vi "pid-toolkit.vi"() -> ()   [LabVIEW 2018, in "pid-toolkit.lvlib"]
uses:
  pid-toolkit.lvlib
  <vilib>/addons/control/pid/autopid.llb/PID autotuning parameters (FO).ctl
  <vilib>/Platform/TimedLoop/XDataNode/timing_clust.ctl
  <vilib>/Platform/TimedLoop/XDataNode/nitl_modes.ctl
  <vilib>/Platform/TimedLoop/XDataNode/wakeup.ctl
  <vilib>/addons/control/pid/pid.llb/PID Advanced (DBL).vi
  <vilib>/platform/TimedLoop/XDataNode/XDataNode.xnode
  <vilib>/Platform/TimedLoop/XDataNode/XDNodeRunTimeDep.lvlib
  <vilib>/addons/control/pid/NI_PID_autopid.lvlib
  <vilib>/addons/control/pid/NI_PID_pid.lvlib
panel:
  out "General Error":errorcluster
  out "Plot":T1(graph)
  out "tuning completed?":bool
  out "plant parameters out":T2={"process gain"=1.0, "time constant (s)"=0.01, "delay time (s)"=0.0} {"delay time (s)" format="%.3f"; "time constant (s)" format="%.3f"; "process gain" format="%.3f"}
  out "PID gains out":T3={"proportional gain (Kc)"=1.0, "integral time (Ti, min)"=0.01, "derivative time (Td, min)"=0.0} {"derivative time (Td, min)" format="%.3f"; "integral time (Ti, min)" format="%.3f"; "proportional gain (Kc)" format="%.3f"}
  in  "reinitialize? (F)":bool
  in  "plant parameters in":T2={"process gain"=1.0, "time constant (s)"=0.01, "delay time (s)"=0.0} {"delay time (s)" format="%.3f"; "time constant (s)" format="%.3f"; "process gain" format="%.3f"}
  in  "PID gains in":T3={"proportional gain (Kc)"=1.0, "integral time (Ti, min)"=0.01, "derivative time (Td, min)"=0.0} {"derivative time (Td, min)" format="%.3f"; "integral time (Ti, min)" format="%.3f"; "proportional gain (Kc)" format="%.3f"}
  in  "output range":cluster{"output high":dbl, "output low":dbl}={"output high"=100.0, "output low"=-100.0} {"output low" format="%.2f"; "output high" format="%.2f"}
  in  "desired temperature":dbl format="%.2f"
  in  "beta":dbl=1.0 format="%.2f"
  in  "autotuning parameters":T4={"type of controller"=0, "time constant factor"=2.0, "step amplitude"=1.0} {"step amplitude" format="%.2f"; "type of controller" items=["P", "PI", "PID"]}
  in  "autotune? (F)":bool
  in  "auto? (T)":bool=TRUE
  in  "alpha":dbl=0.1 format="%.2f"
  out "Output unfiltered":dbl format="%.2f"
  out "Output":u16
  out "High":bool
  out "Low":bool
  in  "Manual":u8(slide) scale=0.0..255.0
  out "Modbus Error":errorcluster
  in  "Off Hook":bool
  in  "Update Rate":dbl caption="Rate"
  out "Failure":bool
  out "Updating":bool
  in  "Update Now":bool
  in  "Maximum":sgl
  in  "Minimum":sgl
  out "Thermometer":sgl(slide) scale=0.0..260.0
  in  "Force exit out of loop":bool
  out "Interval":i64
  out "Duration":i64
  out "Cycle":i32
  in  "Frequency":dbl(slide) scale=0.1..10.0
  # "Loop"
  # "Modbus"
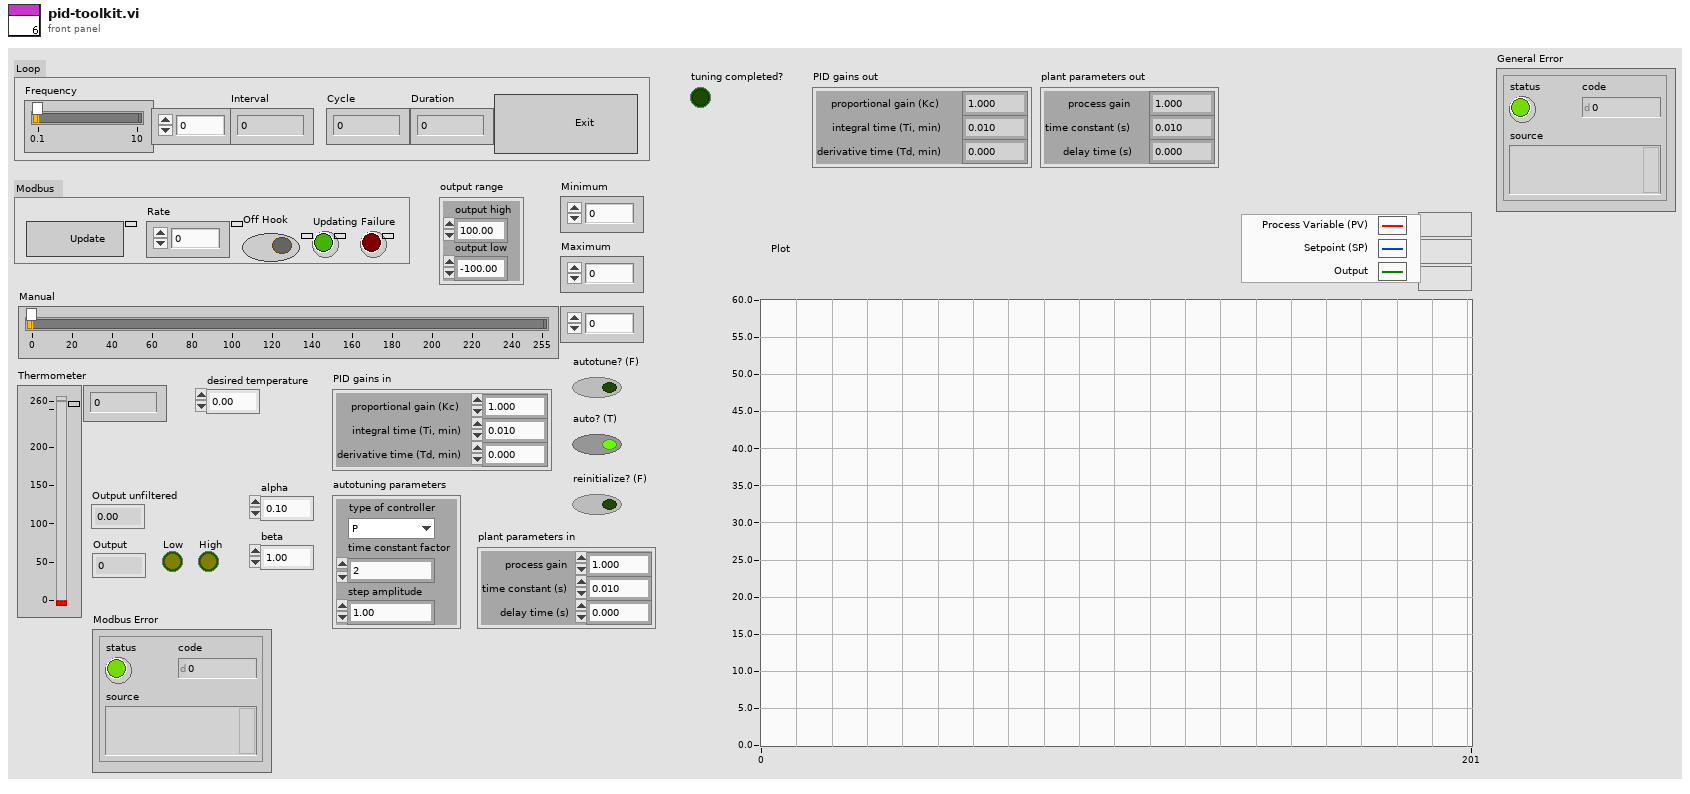
[diagram p1: front panel]
types:
  T1 = cluster{dbl, "desired temperature":dbl, "output":dbl}
  T2 = cluster{"process gain":dbl, "time constant (s)":dbl, "delay time (s)":dbl}
  T3 = cluster{"proportional gain (Kc)":dbl, "integral time (Ti, min)":dbl, "derivative time (Td, min)":dbl}
  T4 = typedef "NI_PID_autopid.lvlib/PID autotuning parameters (FO).ctl" = cluster{"type of controller":u16, "time constant factor":dbl, "step amplitude":dbl}
  T5 = typedef "XDNodeRunTimeDep.lvlib/timing_clust.ctl" = cluster{"Expected End [f-1]":u64, "Actual End [f-1]":u64, "Finished Late? [f-1]":bool, "Expected End [i-1]":u64, "Actual End [i-1]":u64, "Finished Late? [i-1]":bool, "Expected Start [i]":u64, "Actual Start [i]":u64, "Expected Start [f]":u64, "Actual Start [f]":u64, "Source Name":string, "Structure Name":string, "Period":i64, "Deadline":i64, "Offset":i64, "Start":i64, "Priority":i32, "Timeout":i32, "Mode":T6, "Wakeup Reason":T7, "Error":errorcluster, "Source Type":string, "Secondary Source Type":string, "Global End Time":u64, "Global Start Time":u64, "Frame Duration":u64, "Iteration Duration":u64, "Assigned CPU":i32, "I/O Scan Engine Mode":u32}
  T6 = typedef "XDNodeRunTimeDep.lvlib/nitl_modes.ctl" = enum32{"No Change", "Process missed periods, maintain original phase", "Discard missed periods, maintain original phase", "Process missed periods, ignore original phase", "Discard missed periods, ignore original phase"}
  T7 = typedef "XDNodeRunTimeDep.lvlib/wakeup.ctl" = enum32{"Normal", "Aborted", "Asynchronous wakeup", "Timing source error", "Timed loop error", "Timeout"}
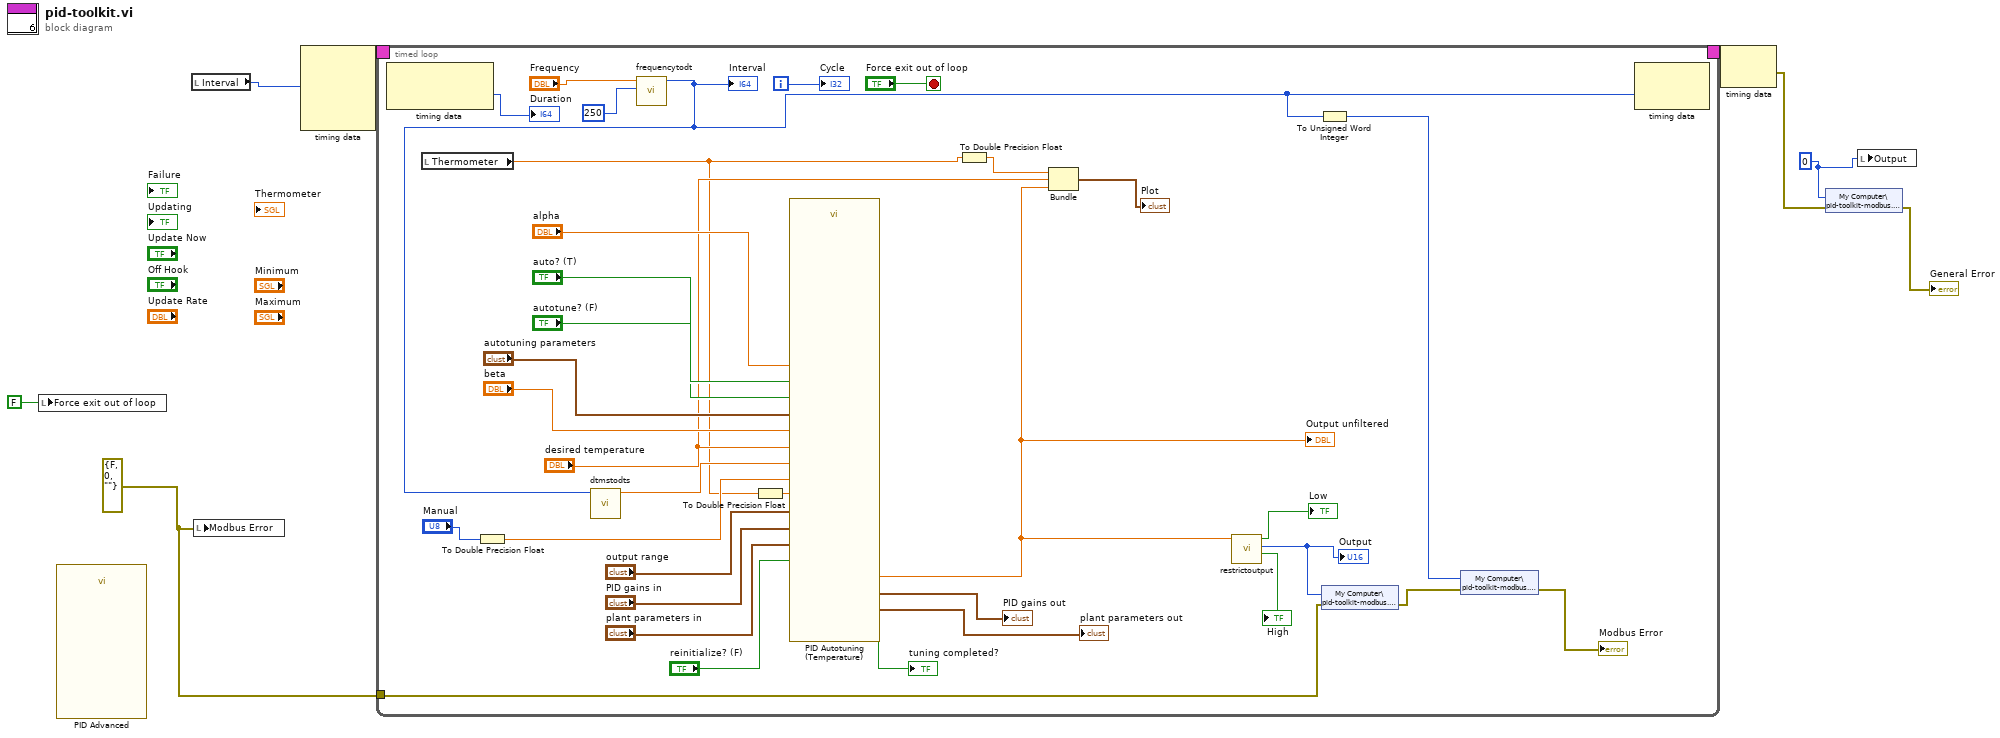
[diagram p0: block diagram]
diagram:
  w2 = u16 0 ("400002")
  w4 = errorcluster {"status"=FALSE, "code"=0, "source"=""} ("Modbus error")
  n1 = local write "Force exit out of loop"(FALSE ("Force exit out of loop")) -> ()
  n2 = call-poly <vilib>:"PID Advanced.vi"() -> ()  [unwired: 14 in, 2 out]
  n3 = local read "Interval"() -> (w5:i64)
  n4 = local write "Modbus Error"(w4) -> ()
  n5 = node-c288(w5) -> (w8:T5)  [unwired: 3 in]
  n6 = timed-loop {
    timing: w8 -> [_]
    timing-out: [_] -> w7
    tunnel: w4 -> [w37]
    i -> [w38]
    stop <- "Force exit out of loop" stop-if-true
    n7 = node-c288() -> (→"Duration":i64)  [unwired: 1 in, 1 out]
    n8 = local read "Thermometer"() -> (w10:sgl)
    n9 = To Double Precision Float(number="Manual") -> (double precision float=w22:dbl)
    n10 = call "frequencytodt.vi"("Default in"=i64 250, "Frequency"="Frequency") -> ("Default out"=w29:i64)  [unwired: 9 in]
    "Interval" <- w29
    n11 = call "dtmstodts.vi"("Default in"=w29) -> ("Numeric"=w23:dbl)  [unwired: 10 in]
    n12 = To Double Precision Float(number=w10) -> (double precision float=w21:dbl)
    n13 = call <vilib>:"PID Autotuning (Temperature).vi"("desired temperature"="desired temperature", "measured temperature"=w21, "plant parameters in"="plant parameters in", "autotune? (F)"="autotune? (F)", "PID gains in"="PID gains in", "dt (s)"=w23, "output range"="output range", "reinitialize? (F)"="reinitialize? (F)", "auto? (T)"="auto? (T)", "beta"="beta", "manual control"=w22, "autotuning parameters"="autotuning parameters", "alpha"="alpha") -> ("output"=w12:dbl, "tuning completed?"=→"tuning completed?":bool, "plant parameters out"=→"plant parameters out":T2, "PID gains out"=→"PID gains out":T3)  [unwired: 3 in]
    "Output unfiltered" <- w12
    n14 = To Double Precision Float(number=w10) -> (double precision float=w13:dbl)
    n15 = Bundle(w13, "desired temperature"="desired temperature", "output"=w12) -> (→"Plot":T1)  [unwired: 1 in]
    n16 = call "restrictoutput.vi"("Input"=w12) -> ("Hig"=→"High":bool, "Output"=w33:u16, "Low"=→"Low":bool)  [unwired: 8 in]
    "Output" <- w33
    n17 = To Unsigned Word Integer(number=w29) -> (unsigned 16bit integer=w30:u16)
    n18 = shared-variable "My Computer\\pid-toolkit-modbus.lvlib\\400002"(w33, error in=w37) -> (error out=w32:errorcluster)
    n19 = shared-variable "My Computer\\pid-toolkit-modbus.lvlib\\400001"(w30, error in=w32) -> (error out=→"Modbus Error":errorcluster)
    n20 = node-c288(w29) -> ()  [unwired: 1 in, 1 out]
    "Cycle" <- w38
  }
  n21 = node-c288(w7) -> (w3:errorcluster)
  n22 = shared-variable "My Computer\\pid-toolkit-modbus.lvlib\\400002"(w2, error in=w3) -> (error out=→"General Error":errorcluster)
  n23 = local write "Output"(w2) -> ()
